vi "GetTimeNow.vi"() -> (2 "start_time_UNIX":dbl, 3 "start_time_string":string)   [LabVIEW 2014]
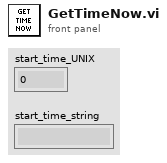
[diagram p1: front panel]
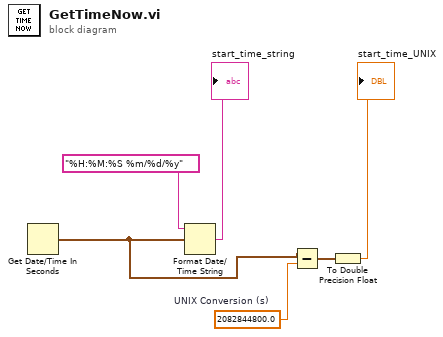
[diagram p0: block diagram]
diagram:
  w3 = 2082844800.0  # UNIX Conversion (s)
  n1 = Get Date/Time In Seconds() -> (seconds since 1Jan1904=w4:timestamp)
  n2 = Format Date/Time String(time format string (%c)="%H:%M:%S %m/%d/%y", seconds (now)=w4) -> (date/time string=→"start_time_string":string)  [unwired: 1 in]
  n3 = Subtract(x=w4, y=w3) -> (x-y=w5:timestamp)
  n4 = To Double Precision Float(number=w5) -> (double precision float=→"start_time_UNIX":dbl)
